vi "JSON TO NUMBER.vi"(7 "IP":string="192.168.23.100", 8 "error in (no error)":errorcluster, 10 "PORT":dbl=1.0 min=1.0 max=4.0 step=1.0, 11 "MASTER":dbl=1.0 min=1.0 max=10.0 step=1.0) -> (0 "error out":errorcluster, 3 "COUNTER":u32 format="%^#.10g")   [LabVIEW 2024]
uses:
  <vilib>/JDP Science/JSONtext/JSONtext.lvlib
  <userlib>/_OpenG.lib/string/string.llb/openg_string.lvlib
panel:
  out "JSON data":string
  # "Non resettable counter data"
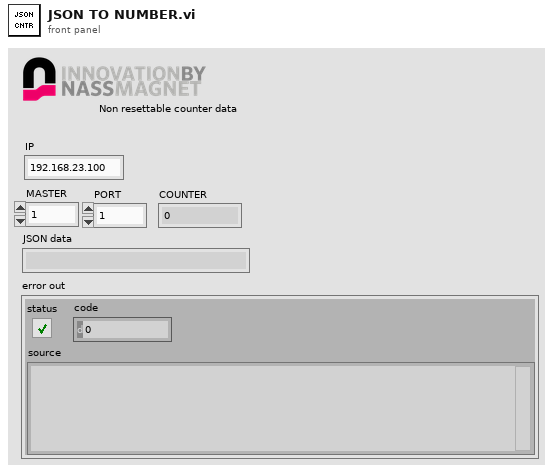
[diagram p1: front panel]
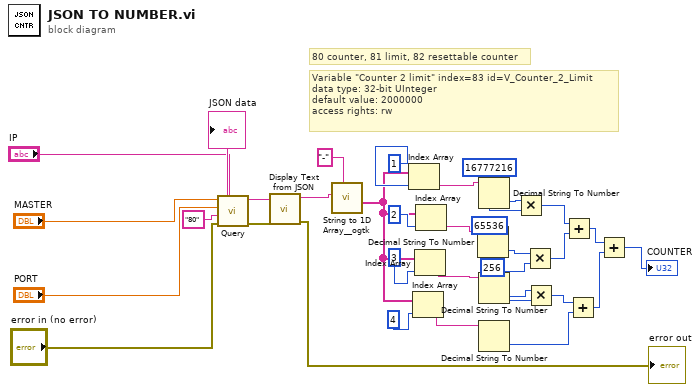
[diagram p0: block diagram]
diagram:
  # "Variable \"Counter 2 limit\" index=83 id=V_Counter_2_Limit\ndata type: 32-bit UInteger\ndefault value: 2000000\naccess rights: rw"
  # "80 counter, 81 limit, 82 resettable counter"
  n1 = call "Query.vi"("IP"="IP", "error in (no error)"="error in (no error)", "PARAMETERS"="80", "PORT"="PORT", "MASTER"="MASTER") -> ("error out"=w19:errorcluster, "JSON data"=w32:string)  [unwired: 5 in]
  "JSON data" <- w32
  n2 = call <vilib>:"Display Text from JSON.vi"("error in (no error)"=w19, "Input JSON"=w32) -> ("error out"=→"error out":errorcluster, "Display Text"=w8:string)  [unwired: 7 in, 1 out]
  n3 = call <userlib>:"String to 1D Array__ogtk.vi"("delimiter (Tab)"="-", "string"=w8) -> ("Array of Strings"=w25:string[])  [unwired: 9 in]
  n4 = Index Array(array=w25, index=1) -> (element=w9:string)
  n5 = Index Array(array=w25, index=4) -> (element=w12:string)
  n6 = Index Array(array=w25, index=3) -> (element=w11:string)
  n7 = Index Array(array=w25, index=2) -> (element=w10:string)
  n8 = Decimal String To Number(string=w10) -> (number=w16:i32)  [unwired: 2 in, 1 out]
  n9 = Decimal String To Number(string=w9) -> (number=w5:i32)  [unwired: 2 in, 1 out]
  n10 = Decimal String To Number(string=w11) -> (number=w1:i32)  [unwired: 2 in, 1 out]
  n11 = Decimal String To Number(string=w12) -> (number=w7:i32)  [unwired: 2 in, 1 out]
  n12 = Multiply(x=w5, y=u32 16777216) -> (x*y=w6:u32)
  n13 = Multiply(x=w16, y=u32 65536) -> (x*y=w13:u32)
  n14 = Multiply(x=w1, y=u32 256) -> (x*y=w14:u32)
  n15 = Add(x=w6, y=w13) -> (x+y=w24:u32)
  n16 = Add(x=w14, y=w7) -> (x+y=w23:u32)
  n17 = Add(x=w24, y=w23) -> (x+y=→"COUNTER":u32)
